vi "Day 5 Puzzle 2.vi"() -> ()   [LabVIEW 2021]
uses:
  <vilib>/Utility/file.llb/Read Delimited Spreadsheet (string).vi
panel:
  out "Result String":string
  out "Final Position":string[][](array[string])
  out "End point":string[](array[string])
  out "Starting point":string[](array[string])
  out "Amount to move":string[](array[string])
  out "Starting point 2":string[](array[string])
  in  "Path":path
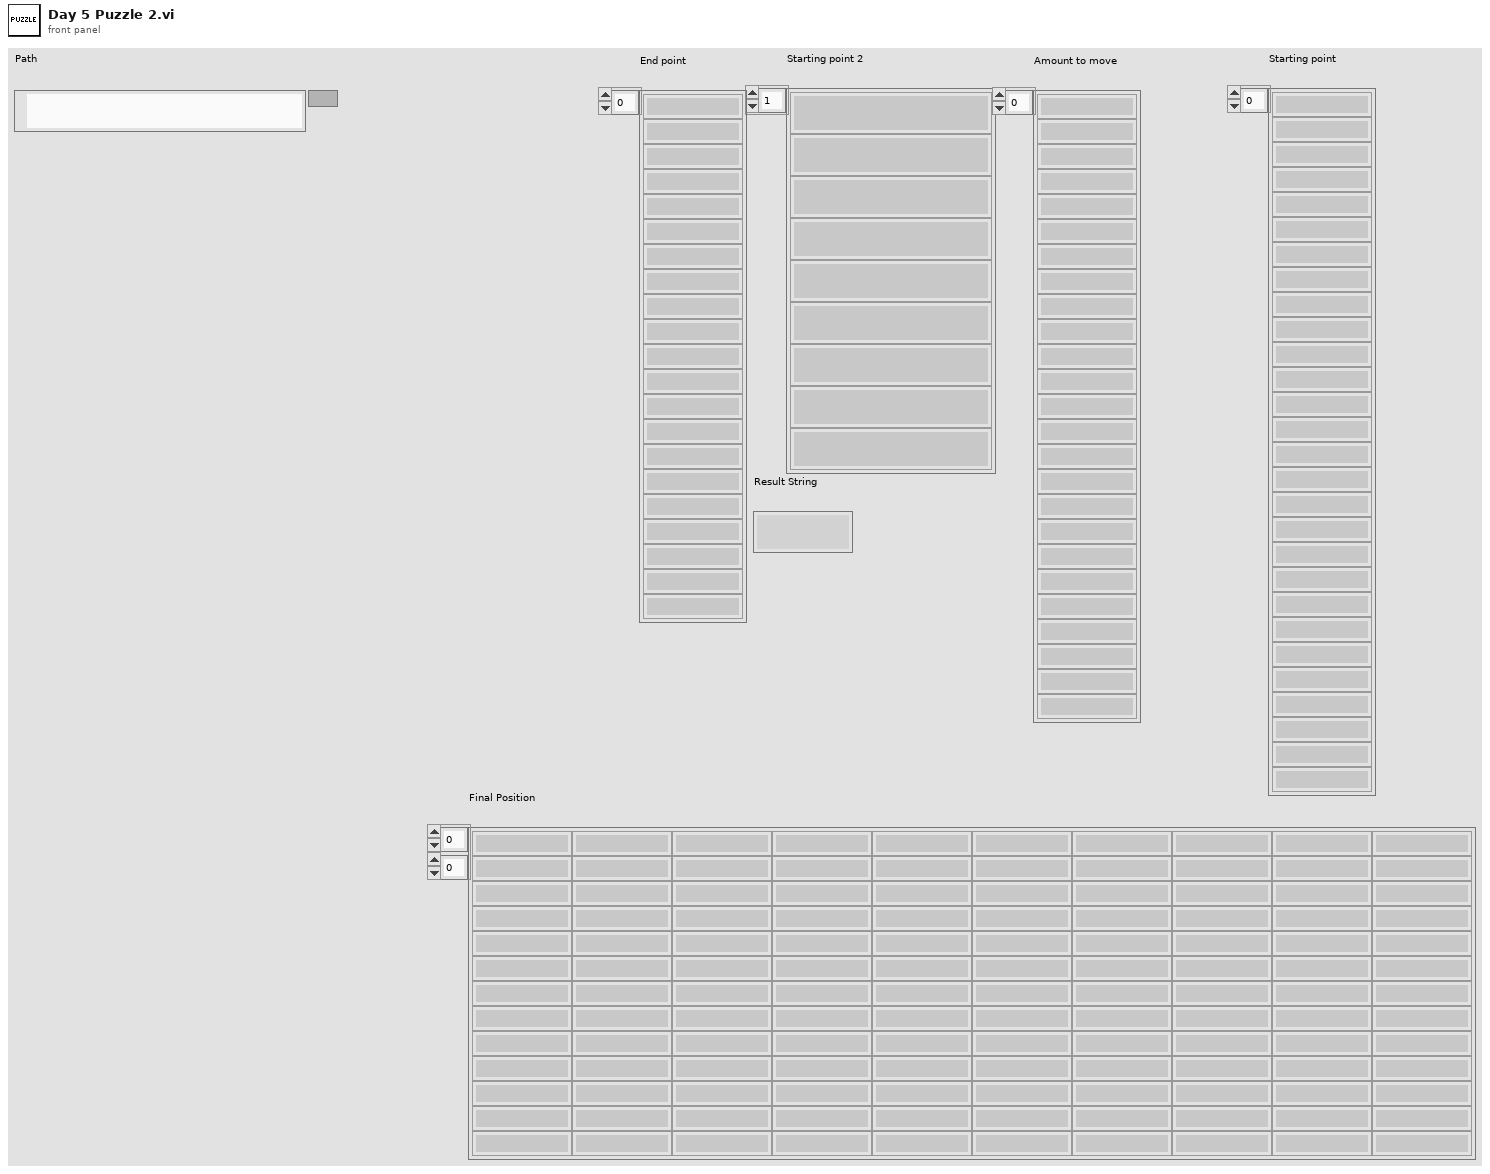
[diagram p1: front panel]
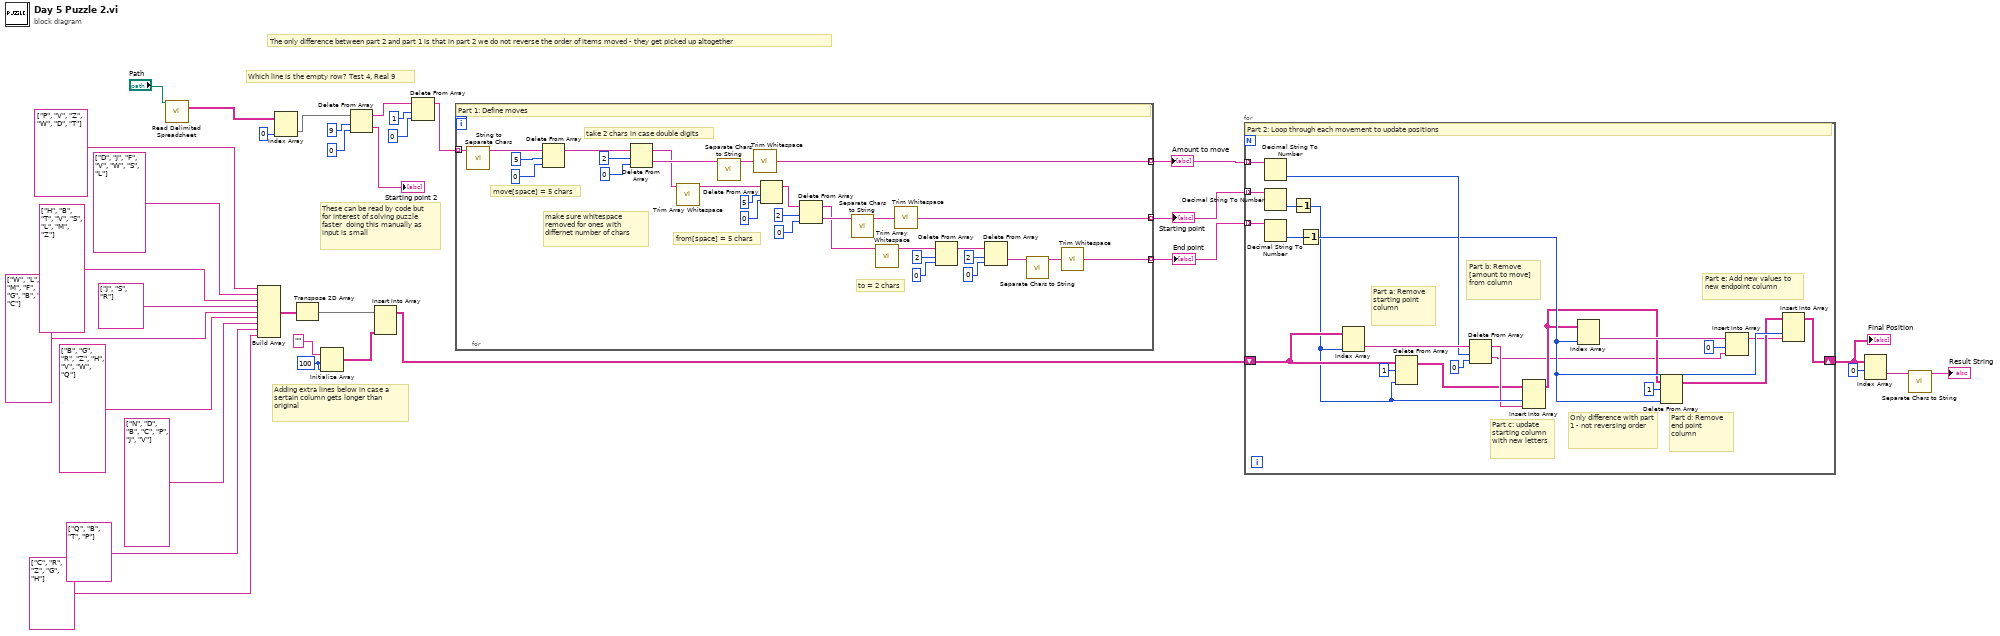
[diagram p0: block diagram]
diagram:
  w11 = 100 ("dimension size")
  # "The only difference between part 2 and part 1 is that in part 2 we do not reverse the order of items moved - they get picked up altogether"
  # "These can be read by code but for interest of solving puzzle faster  doing this manually as input is small"
  # "Adding extra lines below in case a sertain column gets longer than original"
  # "Which line is the empty row? Test 4, Real 9"
  n1 = call-poly <vilib>:"Read Delimited Spreadsheet.vi"("file path (dialog if empty)"="Path") -> ("all rows"=w32:string[][])  [unwired: 9 in, 5 out]
  n2 = Build Array(string[] ["P", "V", "Z", "W", "D", "T"] ("Array 1"), string[] ["D", "J", "F", "V", "W", "S", "L"] ("Array 2"), string[] ["H", "B", "T", "V", "S", "L", "M", "Z"] ("Array 3"), string[] ["J", "S", "R"] ("Array 3"), string[] ["W", "L", "M", "F", "G", "B", "Z", "C"] ("Array 3"), string[] ["B", "G", "R", "Z", "H", "V", "W", "Q"] ("Array 3"), string[] ["N", "D", "B", "C", "P", "J", "V"] ("Array 3"), string[] ["Q", "B", "T", "P"] ("Array 3"), string[] ["C", "R", "Z", "G", "H"] ("Array 3")) -> (w14:string[][])
  n3 = Index Array(array=w32, index (col)=0 ("disabled index (col)")) -> (element=w30:string[])  [unwired: 1 in]
  n4 = Transpose 2D Array(2D array=w14) -> (transposed array=w13:string[][])
  n5 = Initialize Array("", w11, w11) -> (w15:string[][])
  n6 = Delete From Array(array=w30, length=9, index=0) -> (deleted portion=→"Starting point 2":string[], array with subset deleted=w27:string[])
  n7 = Insert Into Array(array=w13, new element=w15) -> (w12:string[][])  [unwired: 2 in]
  n8 = Delete From Array(array=w27, length=1, index=0) -> (array with subset deleted=w23:string[])  [unwired: 1 out]
  n9 = for {
    tunnel: w23 -> [w63] mode=indexing
    tunnel: [w59] -> w19 mode=indexing
    tunnel: [w48] -> w18 mode=indexing
    tunnel: [w38] -> w17 mode=indexing
    # "to = 2 chars"
    # "from[space] = 5 chars"
    # "make sure whitespace \nremoved for ones with differnet number of chars"
    # "take 2 chars in case double digits"
    # "move[space] = 5 chars"
    # "Part 1: Define moves"
    n10 = call "String to Separate Chars.vi"("String"=w63) -> ("Array"=w56:string[])  [unwired: 10 in]
    n11 = Delete From Array(array=w56, length=5, index=0) -> (array with subset deleted=w58:string[])  [unwired: 1 out]
    n12 = Delete From Array(array=w58, length=2, index=0) -> (deleted portion=w47:string[], array with subset deleted=w37:string[])
    n13 = call "Trim Array Whitespace.vi"("Array in"=w37) -> ("Array out"=w36:string[])  [unwired: 10 in]
    n14 = call "Separate Chars to String.vi"("Array"=w47) -> ("String"=w60:string)  [unwired: 10 in]
    n15 = call <vilib>:"Trim Whitespace.vi"("string"=w60) -> ("trimmed string"=w59:string)  [unwired: 1 in]
    n16 = Delete From Array(array=w36, length=5, index=0) -> (array with subset deleted=w46:string[])  [unwired: 1 out]
    n17 = Delete From Array(array=w46, length=2, index=0) -> (deleted portion=w50:string[], array with subset deleted=w35:string[])
    n18 = call "Separate Chars to String.vi"("Array"=w50) -> ("String"=w49:string)  [unwired: 10 in]
    n19 = call "Trim Array Whitespace.vi"("Array in"=w35) -> ("Array out"=w34:string[])  [unwired: 10 in]
    n20 = call <vilib>:"Trim Whitespace.vi"("string"=w49) -> ("trimmed string"=w48:string)  [unwired: 1 in]
    n21 = Delete From Array(array=w34, length=2, index=0) -> (array with subset deleted=w39:string[])  [unwired: 1 out]
    n22 = Delete From Array(array=w39, length=2, index=0) -> (deleted portion=w41:string[])  [unwired: 1 out]
    n23 = call "Separate Chars to String.vi"("Array"=w41) -> ("String"=w40:string)  [unwired: 10 in]
    n24 = call <vilib>:"Trim Whitespace.vi"("string"=w40) -> ("trimmed string"=w38:string)  [unwired: 1 in]
  }
  "Amount to move" <- w19
  "Starting point" <- w18
  "End point" <- w17
  n25 = for {
    tunnel: w19 -> [w85] mode=indexing
    tunnel: w18 -> [w84] mode=indexing
    tunnel: w17 -> [w78] mode=indexing
    shift-right: [w66] -> w10
    shift-left: w12 -> [w74]
    # "Part d: Remove end point column"
    # "Only difference with part 1 - not reversing order"
    # "Part e: Add new values to new endpoint column"
    # "Part c: update starting column with new letters"
    # "Part b: Remove [amount to move] from column"
    # "Part a: Remove starting point column"
    # "Part 2: Loop through each movement to update positions"
    n26 = Decimal String To Number(string=w85) -> (number=w80:i32)  [unwired: 2 in, 1 out]
    n27 = Decimal String To Number(string=w84) -> (number=w83:i32)  [unwired: 2 in, 1 out]
    n28 = Decimal String To Number(string=w78) -> (number=w79:i32)  [unwired: 2 in, 1 out]
    n29 = Decrement(x=w83) -> (x-1=w70:i32)
    n30 = Decrement(x=w79) -> (x-1=w72:i32)
    n31 = Index Array(array=w74, index (col)=w70) -> (element=w82:string[])  [unwired: 1 in]
    n32 = Delete From Array(array=w74, length=1, index (col)=w70) -> (array with subset deleted=w68:string[][])  [unwired: 1 in, 1 out]
    n33 = Delete From Array(array=w82, length=w80, index=0) -> (deleted portion=w65:string[], array with subset deleted=w69:string[])
    n34 = Insert Into Array(array=w68, index (col)=w70, new element=w69) -> (w67:string[][])  [unwired: 1 in]
    n35 = Index Array(array=w67, index (col)=w72) -> (element=w77:string[])  [unwired: 1 in]
    n36 = Delete From Array(array=w67, length=1, index (col)=w72) -> (array with subset deleted=w71:string[][])  [unwired: 1 in, 1 out]
    n37 = Insert Into Array(array=w77, index=0, new element=w65) -> (w64:string[])
    n38 = Insert Into Array(array=w71, index (col)=w72, new element=w64) -> (w66:string[][])  [unwired: 1 in]
  }
  "Final Position" <- w10
  n39 = Index Array(array=w10, index (row)=0) -> (element=w8:string[])  [unwired: 1 in]
  n40 = call "Separate Chars to String.vi"("Array"=w8) -> ("String"=→"Result String":string)  [unwired: 10 in]
